vi "AddLogMsg.vi"(8 "error in (no error)":errorcluster, 10 "LogMessage":string) -> (0 "error out":errorcluster)   [LabVIEW 2017, in "Framework.lvlib"]
uses:
  Framework.lvlib
  Config_class/Config.lvclass/Config.ctl
  Config_class/Read Logging.vi
  Config_class/Config.lvclass
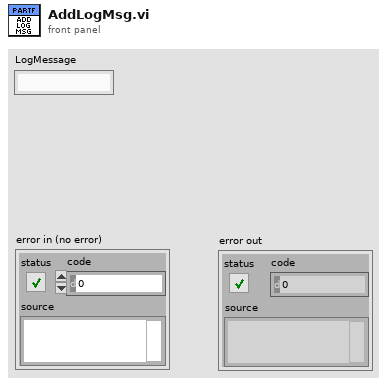
[diagram p1: front panel]
types:
  T1 = typedef "Framework.lvlib/Config.lvclass/Logging.ctl" = cluster{"eLogLvl":T2, "Log File Path":path, "btnLogFile":bool}
  T2 = typedef "Framework.lvlib/Config.lvclass/eLogLvl.ctl" = enum16{"Normal", "Verbose", "None"}
  T3 = enum16{"open", "replace", "create", "open or create", "replace or create", "replace or create with confirmation"}
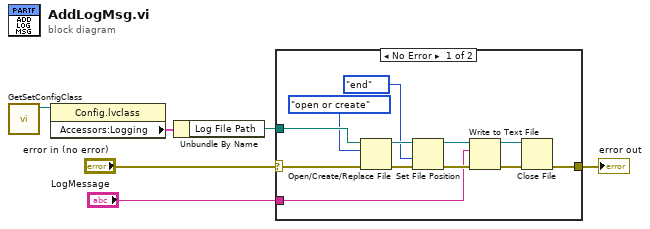
[diagram p0: block diagram]
diagram:
  n1 = call "GetSetConfigClass.vi"() -> ("Ref out"=w3:refnum<class "Config.lvclass">)  [unwired: 11 in]
  n2 = property class="Config.lvclass"(reference=w3) -> ("Accessors:Logging"=w4:T1)  [unwired: 1 in, 2 out]
  n3 = Unbundle By Name(w4) -> ("Log File Path"=w2:path)
  n4 = case shown="No Error" "error in (no error)" {
    selector: "error in (no error)" -> [w18 w19]
    tunnel: "LogMessage" -> [w10 _]
    tunnel: w2 -> [w17 _]
    tunnel: [w7 w19] -> w1
    frame No Error {
      n5 = Open/Create/Replace File(file path (use dialog)=w17, error in=w18, operation (0:open)=T3."open or create") -> (refnum out=w14:refnum<file>, error out=w15:errorcluster)  [unwired: 3 in, 1 out]
      n6 = Set File Position(refnum=w14, from (0:start)=enum16{"start", "end", "current"}."end", error in=w15) -> (refnum out=w12:refnum<file>, error out=w11:errorcluster)  [unwired: 1 in]
      n7 = Write to Text File(file (use dialog)=w12, text=w10, error in=w11) -> (refnum out=w8:refnum<file>, error out=w9:errorcluster)  [unwired: 1 in, 1 out]
      n8 = Close File(refnum=w8, error in=w9) -> (error out=w7:errorcluster)  [unwired: 1 out]
    }
    frame Error {
    }
  }
  "error out" <- w1
